vi "Path-Pick_Next_Tile.vi"(9 "Last Tile":T2, 10 "Adjacent Tiles":T2[](array[typedef]), 11 "Goal":T2) -> (1 "Tile":T1, 2 "New Position":T2)   [LabVIEW 2020]
doc: "<B>Description:</B> Picks the next tile that the maze solver will move to.\nTile Preference: Red >> White >> Purple && Not Previous >> Previous\n\n<B>Date:</B> 05/2019\n<B>Author:</B>Luke Jarocki, Choose Movement Consulting, LLC"
uses:
  Controls/Parse-(X,Y).ctl
  Controls/TileColor.ctl
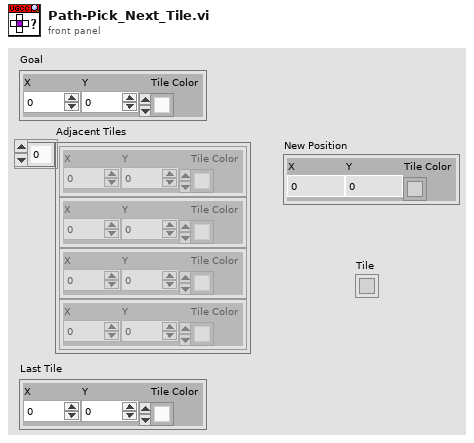
[diagram p1: front panel]
types:
  T1 = typedef "TileColor.ctl" = u16
  T2 = typedef "Parse-(X,Y).ctl" = cluster{"X":i32, "Y":i32, "Tile Color":T1}
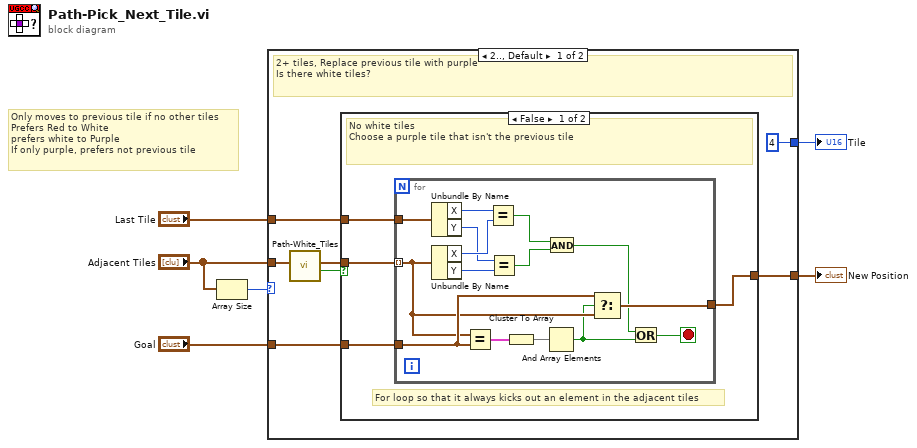
[diagram p0: block diagram]
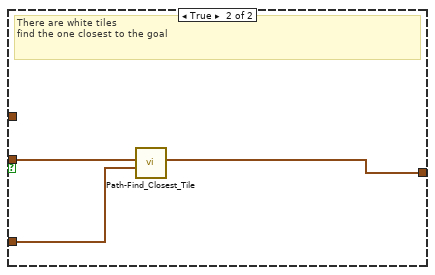
[diagram p2: hidden frame]
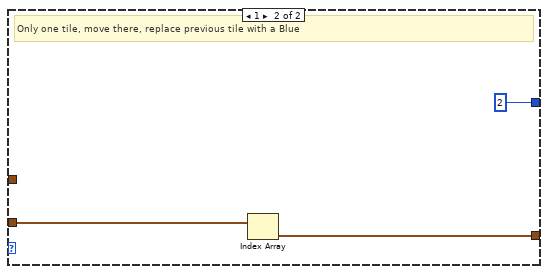
[diagram p3: hidden frame]
diagram:
  # "Only moves to previous tile if no other tiles\nPrefers Red to White\nprefers white to Purple\nIf only purple, prefers not previous tile"
  n1 = Array Size(array="Adjacent Tiles") -> (size(s)=w6:i32)
  n2 = case shown="2.., Default" w6 {
    tunnel: "Adjacent Tiles" -> [w13 w38]
    tunnel: [w9 w37] -> w4
    tunnel: [T1 4 ("Tile") T1 2 ("Tile")] -> w1
    tunnel: "Last Tile" -> [w10 _]
    tunnel: "Goal" -> [w8 _]
    frame 2.., Default {
      # "2+ tiles, Replace previous tile with purple\nIs there white tiles?"
      n3 = call "Path-White_Tiles.vi"("Adjacent Tiles"=w13) -> ("White Tiles?"=w12:bool, "Tiles"=w11:T2[])  [unwired: 9 in]
      n4 = case shown="False" w12 {
        tunnel: w11 -> [w17 w35]
        tunnel: w10 -> [w16 _]
        tunnel: [w15 w34] -> w9
        tunnel: w8 -> [w14 w33]
        frame False {
          # "For loop so that it always kicks out an element in the adjacent tiles"
          # "No white tiles\nChoose a purple tile that isn't the previous tile"
          n5 = for {
            tunnel: w17 -> [w22] mode=indexing
            tunnel: w16 -> [w32]
            tunnel: [w21] -> w15
            tunnel: w14 -> [w23]
            stop <- w18 stop-if-true
            n6 = Unbundle By Name(w32) -> ("X"=w31:i32, "Y"=w29:i32)
            n7 = Unbundle By Name(w22) -> ("X"=w30:i32, "Y"=w28:i32)
            n8 = Equal?(x=w22, y=w23) -> (x = y?=w25:cluster{"X":bool, "Y":bool, "Tile Color":bool})
            n9 = Equal?(x=w31, y=w30) -> (x = y?=w26:bool)
            n10 = Equal?(x=w29, y=w28) -> (x = y?=w27:bool)
            n11 = Cluster To Array(cluster=w25) -> (array=w24:bool[])
            n12 = And Array Elements(Boolean array=w24) -> (logical AND=w19:bool)
            n13 = And(x=w26, y=w27) -> (x .and. y?=w20:bool)
            n14 = Select(t=w23, s=w19, f=w22) -> (s? t:f=w21:T2)
            n15 = Or(x=w20, y=w19) -> (x .or. y?=w18:bool)
          }
        }
        frame True {
          # "There are white tiles\nfind the one closest to the goal"
          n16 = call "Path-Find_Closest_Tile.vi"("Goal"=w33, "Tiles"=w35) -> ("Closest Tile"=w34:T2)  [unwired: 9 in]
        }
      }
    }
    frame 1 {
      # "Only one tile, move there, replace previous tile with a Blue"
      n17 = Index Array(array=w38) -> (element=w37:T2)  [unwired: 1 in]
    }
  }
  "New Position" <- w4
  "Tile" <- w1
